vi "Create Loader String.vi"(11 "Loader Name":string) -> (3 "Loader string":string)   [LabVIEW 2021, in "CIFLogs.lvlib"]
uses:
  CIFLogs.lvlib
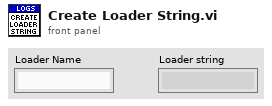
[diagram p1: front panel]
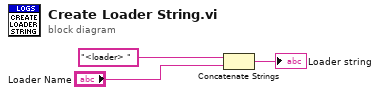
[diagram p0: block diagram]
diagram:
  n1 = Concatenate Strings("<loader> " ("string"), "Loader Name") -> (→"Loader string":string)
